vi "CorWFM.vi"(6 "Index":i8, 8 "error in (no error)":errorcluster, 9 "Sampling Length":sgl[unit]=0.055, 10 "Sampling Frequency":sgl[unit]=55.0, 11 "Cohorts in":refnum<class "Cohort.lvclass">[](array[class])) -> (0 "error out":errorcluster)   [LabVIEW 2012, in "Cohort.lvclass"]
uses:
  Cohort.lvclass
  CorWFMPanel.ctl
  StimulCtrls.lvlib
panel:
  in  "Cohort List":i32(listbox)
  in  "X-Axis Time":cluster{sgl, sgl}(slide)={2.0105264, 0.9157895} scale=-1.0..3.0
  in  "Exit":bool
  in  "Y-axis Amplitude":cluster{sgl, sgl}(slide)={1.0315789, 0.021052632} scale=-2.0..10.0
  out "Electrode Set":T1
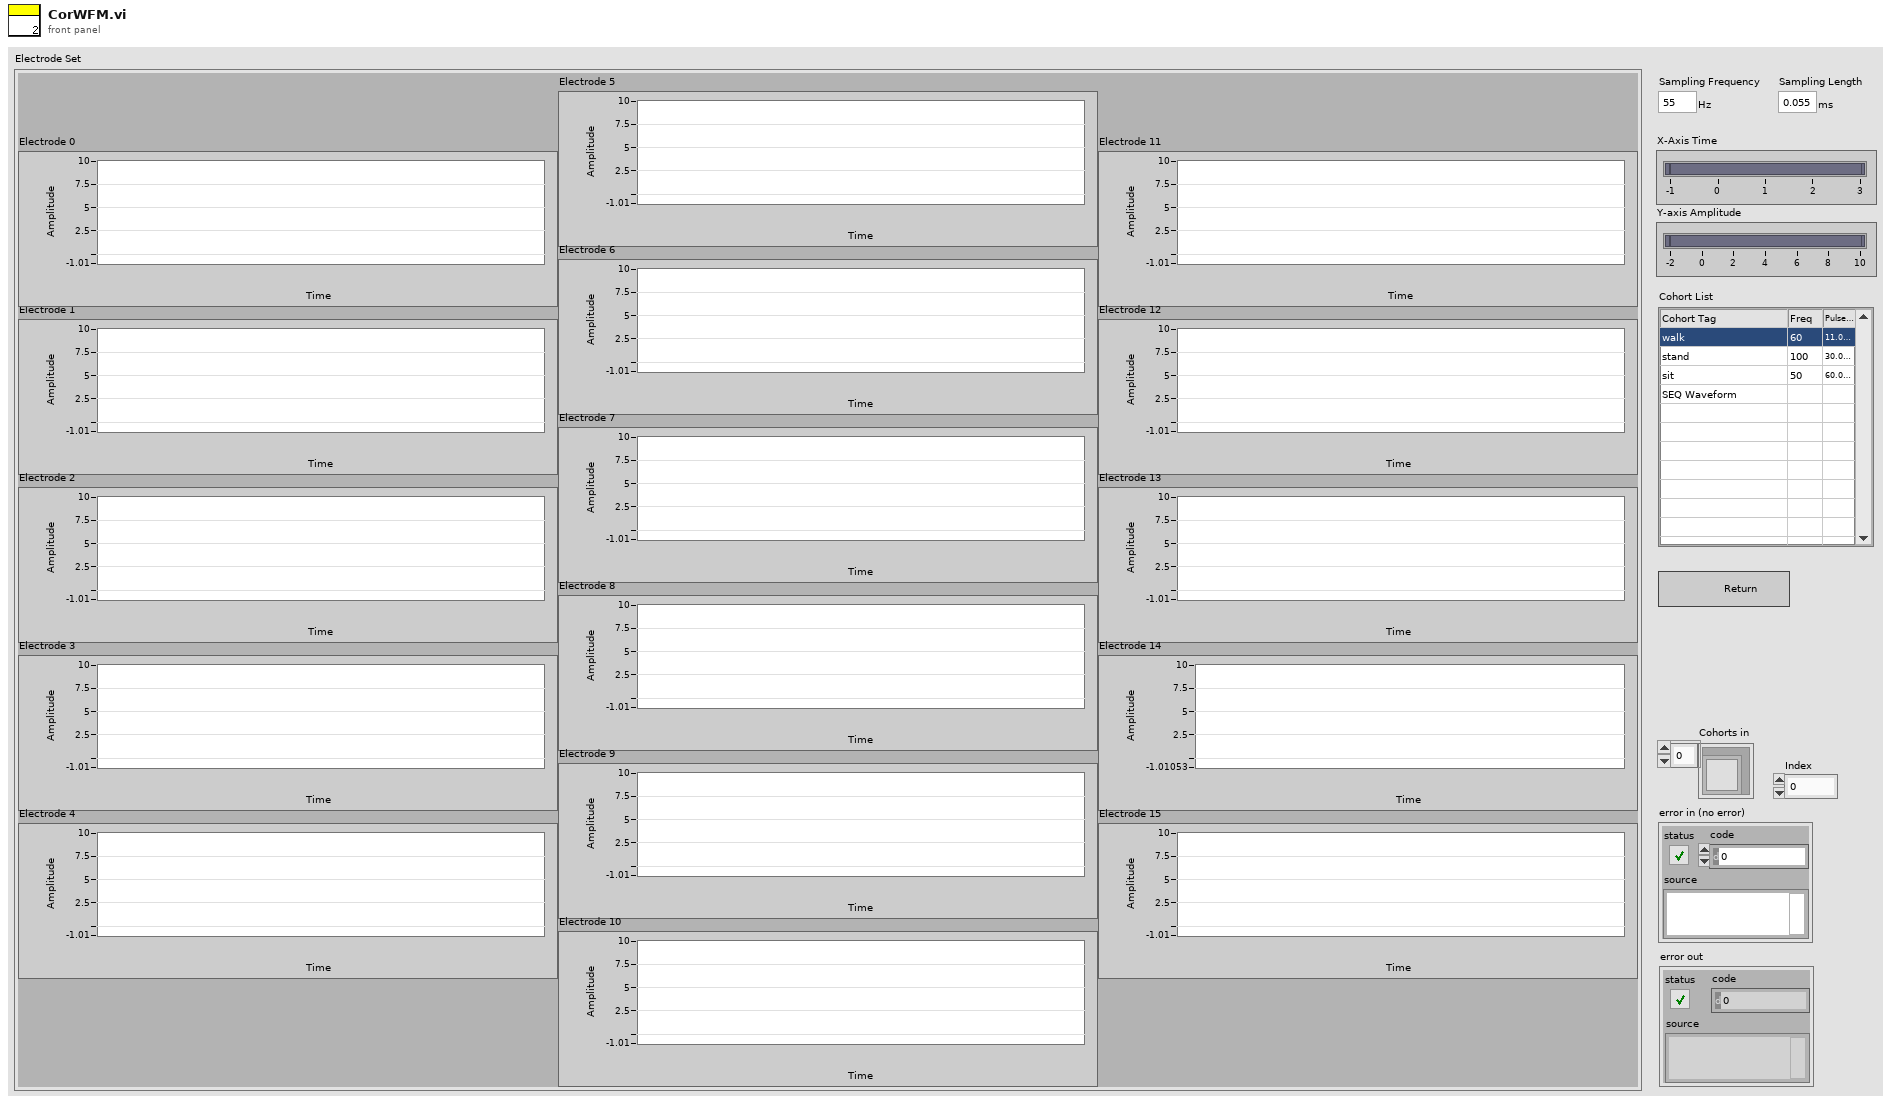
[diagram p1: front panel]
types:
  T1 = typedef "StimulCtrls.lvlib/CorWFMPanel.ctl" = cluster{"Electrode 0":dbl[], "Electrode 1":dbl[], "Electrode 2":dbl[], "Electrode 3":dbl[], "Electrode 4":dbl[], "Electrode 5":dbl[], "Electrode 6":dbl[], "Electrode 7":dbl[], "Electrode 8":dbl[], "Electrode 9":dbl[], "Electrode 10":dbl[], "Electrode 11":dbl[], "Electrode 12":dbl[], "Electrode 13":dbl[], "Electrode 14":dbl[], "Electrode 15":dbl[]}
  T2 = enum16{"UpdateWFM", "AxisAdjust", "Wait", "Exit"}
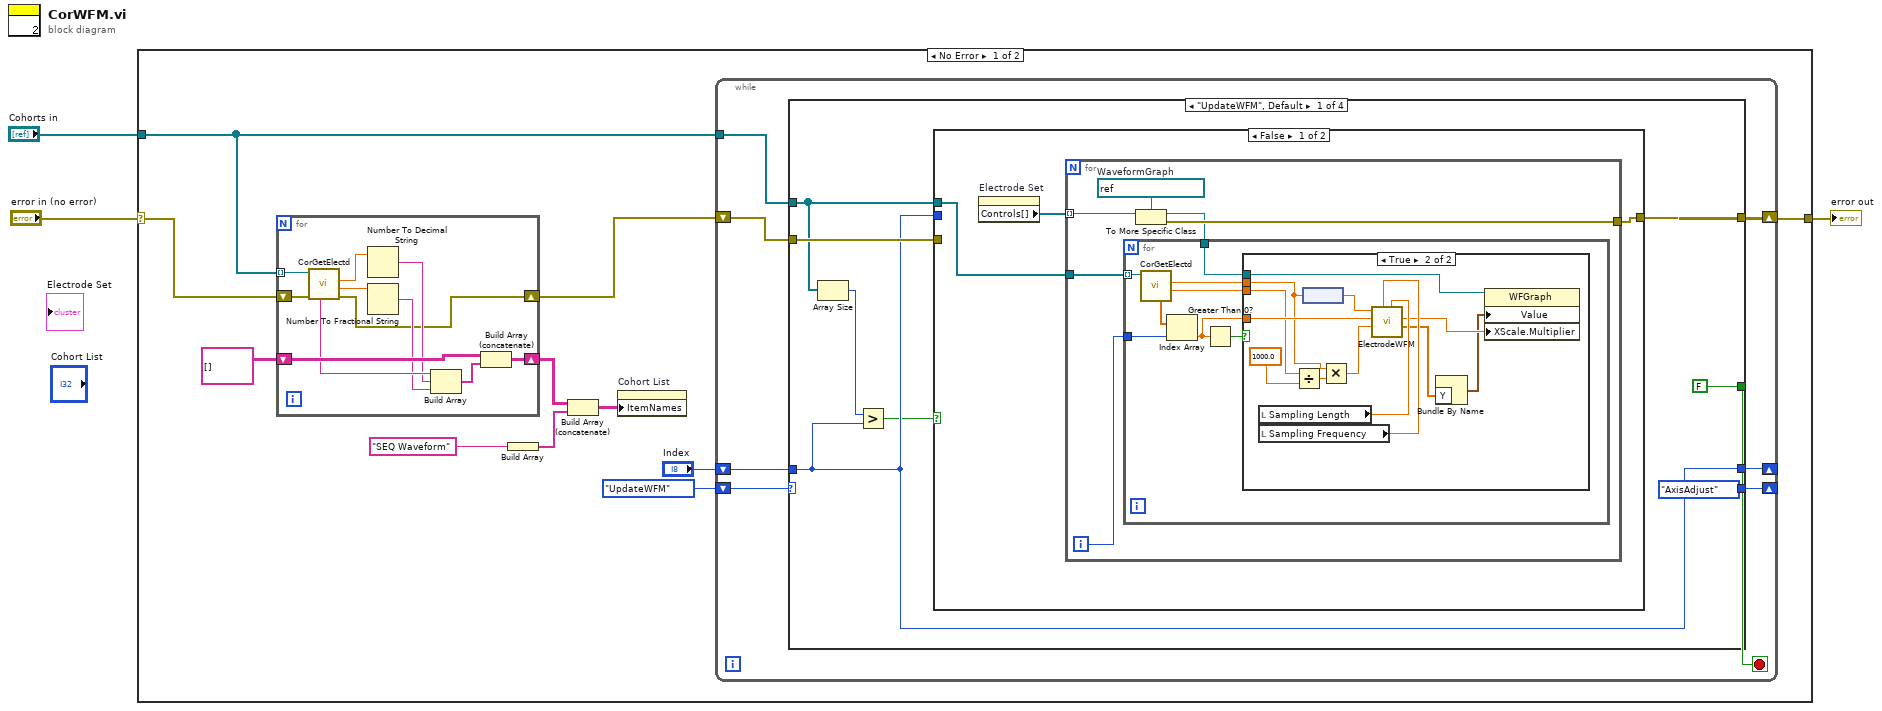
[diagram p0: block diagram]
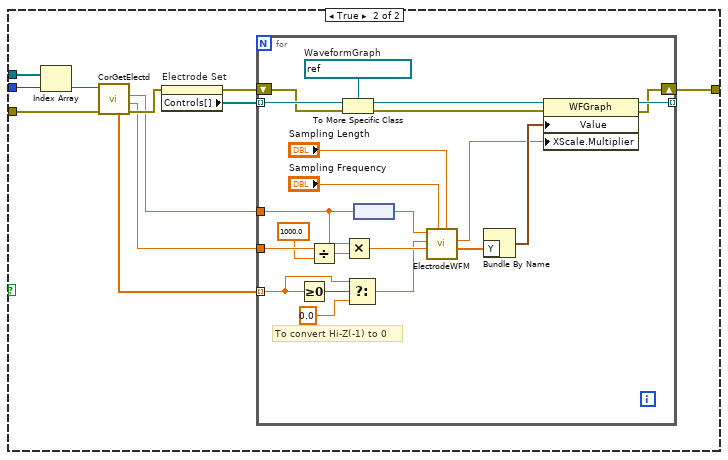
[diagram p3: hidden frame]
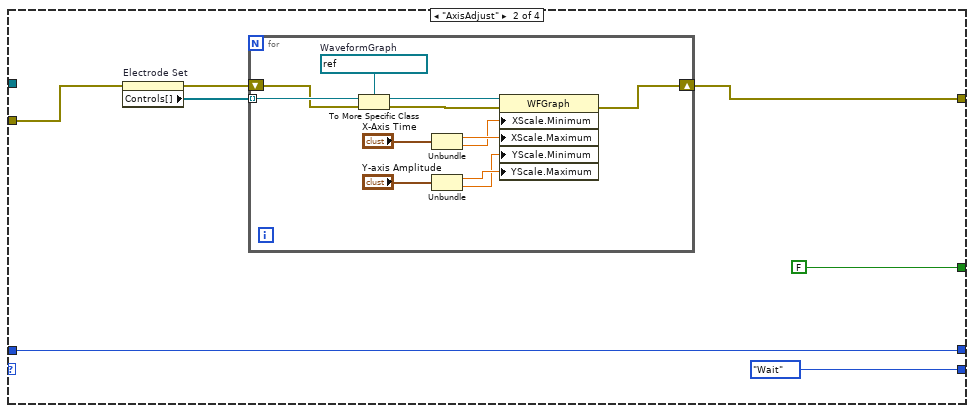
[diagram p4: hidden frame]
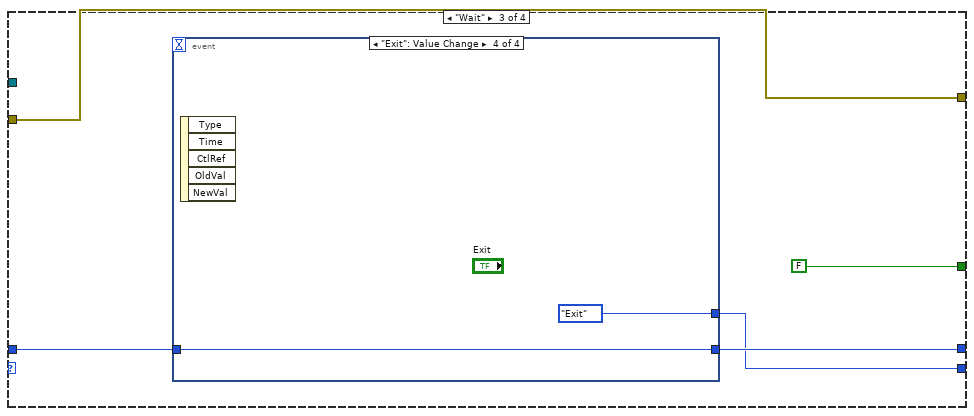
[diagram p5: hidden frame]
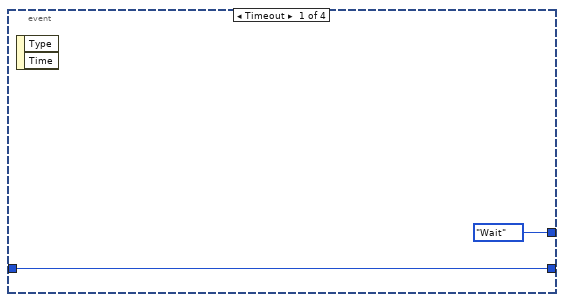
[diagram p6: hidden frame]
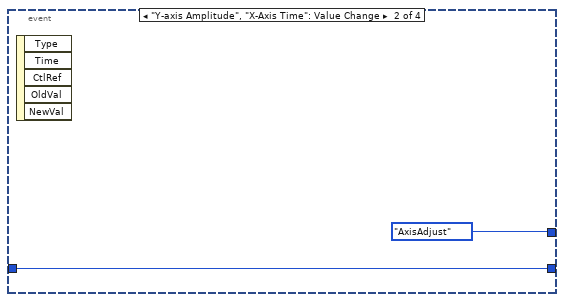
[diagram p7: hidden frame]
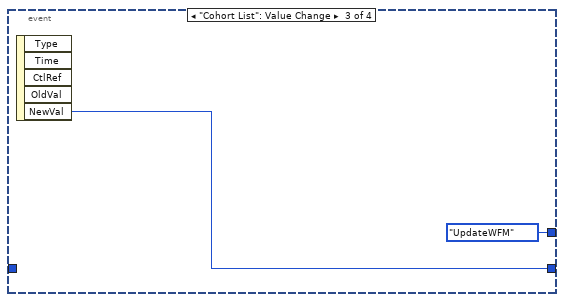
[diagram p8: hidden frame]
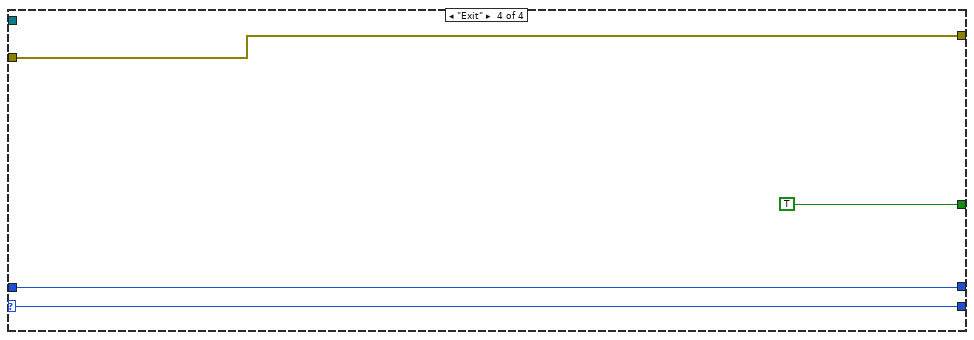
[diagram p9: hidden frame]
diagram:
  n1 = case shown="No Error" "error in (no error)" {
    selector: "error in (no error)" -> [w8 w141]
    tunnel: [w4 w141] -> w2
    tunnel: "Cohorts in" -> [w9 _]
    frame No Error {
      n2 = for {
        tunnel: w9 -> [w140] mode=indexing
        shift-right: [w139] -> w12
        shift-left: string[][] [] -> [w138]
        shift-right: [w130] -> w5
        shift-left: w8 -> [w131]
        n3 = call-dynamic "CorGetElectd.vi"("error in (no error)"=w131, "Cohort in"=w140) -> ("error out"=w130:errorcluster, "Pulse Width [ms]"=w133:sgl, "Pulse Frequency [Hz]"=w135:sgl, "COR Tag"=w136:string)  [unwired: 5 in, 1 out]
        n4 = Number To Decimal String(number=w135) -> (decimal integer string=w134:string)  [unwired: 1 in]
        n5 = Number To Fractional String(number=w133) -> (F-format string=w132:string)  [unwired: 3 in]
        n6 = Build Array(w136, w134, w132) -> (w137:string[])
        n7 = Build Array (concatenate)(w138, w137) -> (w139:string[][])
      }
      n8 = Build Array("SEQ Waveform") -> (w10:string[])
      n9 = Build Array (concatenate)(w12, w10) -> (w11:string[][])
      n10 = property on="Cohort List" class="MCListbox (strict)"("ItemNames"=w11) -> ()  [unwired: 2 in, 2 out]
      n11 = while {
        tunnel: w9 -> [w22]
        shift-right: [w19] -> _
        shift-left: T2."UpdateWFM" -> [w21]
        shift-right: [w18] -> _
        shift-left: "Index" -> [w20]
        shift-right: [w16] -> w4
        shift-left: w5 -> [w17]
        stop <- w15 stop-if-true
        n12 = case shown="\"UpdateWFM\", Default" w21 {
          selector: w21 -> [_ _ _ w127]
          tunnel: w22 -> [w26 _ _ _]
          tunnel: w20 -> [w24 w99 w117 w128]
          tunnel: [enum16{"UpdateWFM", "AxisAdjust", "Wait"}."AxisAdjust" enum16{"UpdateWFM", "AxisAdjust", "Wait"}."Wait" w115 w127] -> w19
          tunnel: [w24 w99 w116 w128] -> w18
          tunnel: [w28 w95 w114 w126] -> w16
          tunnel: w17 -> [w29 w97 w114 w126]
          tunnel: [FALSE ("Exit") FALSE ("Exit") FALSE ("Exit") TRUE ("Exit")] -> w15
          frame "UpdateWFM", Default {
            n13 = Array Size(array=w26) -> (size(s)=w25:i32)
            n14 = Greater?(x=w25, y=w24) -> (0:w23:bool)
            n15 = case shown="False" w23 {
              tunnel: w29 -> [_ w64]
              tunnel: [w31 w63] -> w28
              tunnel: w26 -> [w32 w62]
              tunnel: w24 -> [_ w61]
              frame False {
                n16 = property on="Electrode Set" class="Clust (strict)"() -> ("Controls[]"=w33:refnum<vi>[])  [unwired: 2 in, 2 out]
                n17 = for {
                  tunnel: w33 -> [w38] mode=indexing
                  tunnel: w32 -> [w37]
                  tunnel: [w35] -> w31
                  i -> [w36]
                  w39 = refnum<vi> refnum  # WaveformGraph
                  n18 = To More Specific Class(target class=w39, reference=w38) -> (specific class reference=w34:refnum<vi>, error out=w35:errorcluster)  [unwired: 1 in]
                  n19 = for {
                    tunnel: w37 -> [w47] mode=indexing
                    tunnel: w36 -> [w45]
                    tunnel: w34 -> [w40]
                    n20 = call-dynamic "CorGetElectd.vi"("Cohort in"=w47) -> ("Pulse Width [ms]"=w42:sgl, "Pulse Frequency [Hz]"=w43:sgl, "Amplitude"=w46:sgl[])  [unwired: 6 in, 2 out]
                    n21 = Index Array(array=w46, index=w45) -> (element=w41:sgl)
                    n22 = Greater Than 0?(x=w41) -> (x > 0?=w44:bool)
                    n23 = case shown="True" w44 {
                      tunnel: w43 -> [_ w55]
                      tunnel: w42 -> [_ w56]
                      tunnel: w41 -> [_ w59]
                      tunnel: w40 -> [_ w50]
                      frame False {
                      }
                      frame True {
                        n24 = local read "Sampling Length"() -> (w53:sgl[unit])
                        n25 = local read "Sampling Frequency"() -> (w52:sgl[unit])
                        n26 = Divide(x=w56, y=sgl 1000.0) -> (x/y=w58:sgl)
                        n27 = node(w55) -> (w60:sgl[unit])
                        n28 = Multiply(x=w55, y=w58) -> (x*y=w54:sgl)
                        n29 = call "ElectrodeWFM.vi"("Sampling Length"=w53, "Sampling Freq"=w52, "Pulse Width Ratio"=w54, "Pulse Amplitude"=w59, "Pulse Freq"=w60) -> ("Signal Array"=w49:dbl[], "dt [s]"=w51:dbl)  [unwired: 4 in, 1 out]
                        n30 = Bundle By Name("Y"=w49) -> (w48:waveform(dbl))  [unwired: 1 in]
                        n31 = property class="WFGraph"(reference=w50, "Value"=w48, "XScale.Multiplier"=w51) -> ()  [unwired: 1 in, 2 out]
                      }
                    }
                  }
                }
              }
              frame True {
                n32 = Index Array(array=w62, index=w61) -> (element=w65:refnum<class "Cohort.lvclass">)
                n33 = call-dynamic "CorGetElectd.vi"("error in (no error)"=w64, "Cohort in"=w65) -> ("error out"=w70:errorcluster, "Pulse Width [ms]"=w68:sgl, "Pulse Frequency [Hz]"=w69:sgl, "Amplitude"=w66:sgl[])  [unwired: 5 in, 1 out]
                n34 = property on="Electrode Set" class="Clust (strict)"(error in=w70) -> (error out=w67:errorcluster, "Controls[]"=w71:refnum<vi>[])  [unwired: 1 in, 1 out]
                n35 = for {
                  tunnel: w71 -> [w93] mode=indexing
                  tunnel: w66 -> [w80] mode=indexing
                  tunnel: w69 -> [w89]
                  tunnel: w68 -> [w88]
                  tunnel: [w77] -> _ mode=indexing
                  shift-right: [w72] -> w63
                  shift-left: w67 -> [w82]
                  w76 = refnum<vi> refnum  # WaveformGraph
                  # "To convert Hi-Z(-1) to 0"
                  n36 = Greater Or Equal To 0?(x=w80) -> (x >= 0?=w81:bool)
                  n37 = Divide(x=w88, y=sgl 1000.0) -> (x/y=w87:sgl)
                  n38 = To More Specific Class(target class=w76, reference=w93, error in=w82) -> (specific class reference=w92:refnum<vi>, error out=w91:errorcluster)
                  n39 = Multiply(x=w89, y=w87) -> (x*y=w85:sgl)
                  n40 = Select(t=w80, s=w81, f=sgl 0.0) -> (s? t:f=w78:sgl)
                  n41 = node(w89) -> (w90:sgl[unit])
                  n42 = call "ElectrodeWFM.vi"("Sampling Length"="Sampling Length", "Sampling Freq"="Sampling Frequency", "Pulse Width Ratio"=w85, "Pulse Amplitude"=w78, "Pulse Freq"=w90) -> ("Signal Array"=w75:dbl[], "dt [s]"=w73:dbl)  [unwired: 4 in, 1 out]
                  n43 = Bundle By Name("Y"=w75) -> (w74:waveform(dbl))  [unwired: 1 in]
                  n44 = property class="WFGraph"(reference=w92, error in=w91, "Value"=w74, "XScale.Multiplier"=w73) -> (reference out=w77:refnum<vi>, error out=w72:errorcluster)
                }
              }
            }
          }
          frame "AxisAdjust" {
            n45 = property on="Electrode Set" class="Clust (strict)"(error in=w97) -> (error out=w96:errorcluster, "Controls[]"=w100:refnum<vi>[])  [unwired: 1 in, 1 out]
            n46 = for {
              tunnel: w100 -> [w103] mode=indexing
              shift-right: [w102] -> w95
              shift-left: w96 -> [w101]
              w106 = refnum<vi> refnum  # WaveformGraph
              n47 = To More Specific Class(target class=w106, reference=w103, error in=w101) -> (specific class reference=w105:refnum<vi>, error out=w104:errorcluster)
              n48 = Unbundle("X-Axis Time") -> (w110:sgl, w109:sgl)
              n49 = Unbundle("Y-axis Amplitude") -> (w108:sgl, w107:sgl)
              n50 = property class="WFGraph"(reference=w105, error in=w104, "XScale.Minimum"=w109, "XScale.Maximum"=w110, "YScale.Minimum"=w107, "YScale.Maximum"=w108) -> (error out=w102:errorcluster)  [unwired: 1 out]
            }
          }
          frame "Wait" {
            n51 = event shown="[3] \"Exit\": Value Change" {
              selector: _ -> [_ _ _ _]
              dyn-events: _ -> [_ _ _ _]
              timeout: _ -> [_ _ _ _]
              tunnel: w117 -> [w119 w121 _ w125]
              tunnel: [w119 w121 w123 w125] -> w116
              tunnel: [enum16{"UpdateWFM", "AxisAdjust", "Wait"}."Wait" enum16{"UpdateWFM", "AxisAdjust", "Wait"}."AxisAdjust" enum16{"UpdateWFM", "AxisAdjust", "Wait"}."UpdateWFM" T2."Exit"] -> w115
              event Timeout {
                n52 = event-data() -> ()  [unwired: 1 in, 2 out]
              }
              event "Y-axis Amplitude", "X-Axis Time": Value Change {
                n53 = event-data() -> ()  [unwired: 1 in, 5 out]
              }
              event "Cohort List": Value Change {
                n54 = event-data() -> ("NewVal"=w123:i32)  [unwired: 1 in, 4 out]
              }
              event "Exit": Value Change {
                n55 = event-data() -> ()  [unwired: 1 in, 5 out]
              }
            }
          }
          frame "Exit" {
          }
        }
      }
    }
    frame Error {
    }
  }
  "error out" <- w2
